vi "Field Info to Cluster Item Info.vi"   [LabVIEW 2021]
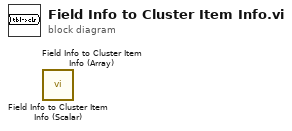
[diagram p0: block diagram]
diagram:
  n1 = call "Field Info to Cluster Item Info (Scalar).vi"() -> ()  [unwired: 1 in, 1 out]
  n2 = call "Field Info to Cluster Item Info (Array).vi"() -> ()  [unwired: 1 in, 1 out]
